vi "Integration Frequency Domain (1 Ch Wfm).vi"(8 "Highpass Cutoff":dbl, 9 "Conversion Scale Factor":sgl, 10 "Conversion Op":T1, 11 "Waveform":waveform(sgl)) -> (3 "Integrated Waveform":waveform(sgl))   [LabVIEW 2017, in "VibrationAnalysisFunctions.lvlib"]
uses:
  <vilib>/addons/InsightCM/Utilities/Analysis/Vibration/VibrationAnalysisFunctions.lvlib
  <vilib>/addons/InsightCM/Utilities/Analysis/Shared/controls/ConversionOp.ctl
  <vilib>/Analysis/2dsp.llb/Real FFT.vi
  <vilib>/Analysis/2dsp.llb/Inverse Real FFT.vi
  <vilib>/Analysis/NI_AALPro.lvlib
  <vilib>/addons/InsightCM/Utilities/Analysis/Shared/AnalysisHelper.lvlib
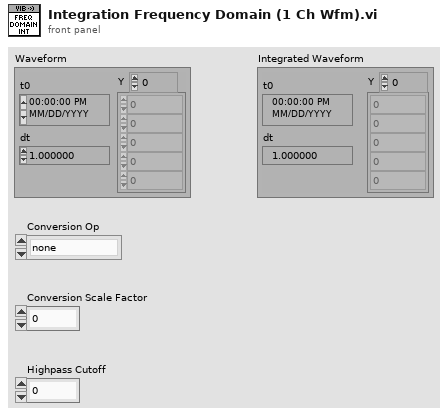
[diagram p1: front panel]
types:
  T1 = typedef "AnalysisHelper.lvlib/ConversionOp.ctl" = enum16{"none", "singleInt", "doubleInt", "singleDiff", "doubleDiff"}
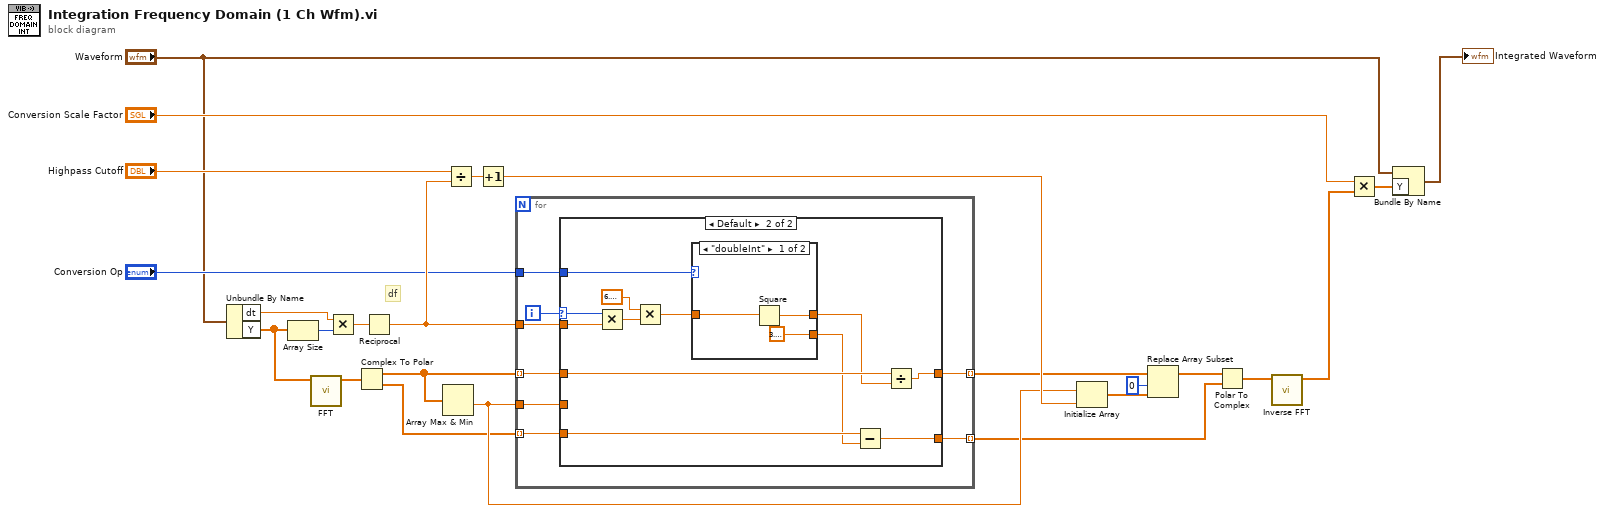
[diagram p0: block diagram]
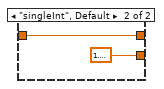
[diagram p3: hidden frame]
diagram:
  # "df"
  n1 = Unbundle By Name("Waveform") -> ("dt"=w13:dbl, "Y"=w6:sgl[])
  n2 = Array Size(array=w6) -> (size(s)=w12:i32)
  n3 = call-poly <vilib>:"FFT.vi"("X"=w6) -> ("FFT {X}"=w4:cdb[])  [unwired: 9 in, 1 out]
  n4 = Multiply(x=w13, y=w12) -> (x*y=w14:dbl)
  n5 = Complex To Polar(r * e^(i*theta)=w4) -> (r=w5:dbl[], theta=w7:dbl[])
  n6 = Reciprocal(x=w14) -> (1/x=w22:dbl)
  n7 = Array Max & Min(array=w5) -> (min value=w18:dbl)  [unwired: 3 out]
  n8 = Divide(x="Highpass Cutoff", y=w22) -> (x/y=w23:dbl)
  n9 = Increment(x=w23) -> (x+1=w24:dbl)
  n10 = for {
    tunnel: w5 -> [w32] mode=indexing
    tunnel: w18 -> [w30]
    tunnel: [w29] -> w16 mode=indexing
    tunnel: "Conversion Op" -> [w28]
    tunnel: w7 -> [w27] mode=indexing
    tunnel: [w26] -> w8 mode=indexing
    tunnel: w22 -> [w25]
    i -> [w31]
    n11 = case shown="Default" w31 {
      selector: w31 -> [_ w44]
      tunnel: w32 -> [_ w46]
      tunnel: w30 -> [w34 _]
      tunnel: [w34 w35] -> w29
      tunnel: w28 -> [_ w45]
      tunnel: w27 -> [w33 w43]
      tunnel: [w33 w41] -> w26
      tunnel: w25 -> [_ w40]
      frame 0 {
      }
      frame Default {
        n12 = Multiply(x=w44, y=w40) -> (x*y=w39:dbl)
        n13 = Multiply(x=6.283185307179586, y=w39) -> (x*y=w37:dbl)
        n14 = case shown="\"doubleInt\"" w45 {
          tunnel: [3.141592653589793 1.5707963267948966] -> w42
          tunnel: w37 -> [w48 w50]
          tunnel: [w47 w50] -> w36
          frame "doubleInt" {
            n15 = Square(x=w48) -> (x^2=w47:dbl)
          }
          frame "singleInt", Default {
          }
        }
        n16 = Subtract(x=w43, y=w42) -> (x-y=w41:dbl)
        n17 = Divide(x=w46, y=w36) -> (x/y=w35:dbl)
      }
    }
  }
  n18 = Initialize Array(w18, w24) -> (w19:dbl[])
  n19 = Replace Array Subset(array=w16, new element=w19, index=0) -> (w17:dbl[])
  n20 = Polar To Complex(1:w8, 2:w17) -> (0:w9:cdb[])
  n21 = call-poly <vilib>:"Inverse FFT.vi"("FFT {X}"=w9) -> ("X"=w11:dbl[])  [unwired: 9 in, 1 out]
  n22 = Multiply(x="Conversion Scale Factor", y=w11) -> (x*y=w2:dbl[])
  n23 = Bundle By Name(cluster="Waveform", "Y"=w2) -> (→"Integrated Waveform":waveform(sgl))
